vi "DeleteRecord.vi"(0 "reference in":refnum<class "CustomersData.lvclass">, 2 "Customer":string, 5 "error in (no error)":errorcluster) -> (14 "reference out":refnum<class "CustomersData.lvclass">, 19 "error out":errorcluster)   [LabVIEW 2020, in "CustomersData.lvclass"]
uses:
  CustomersData.lvclass
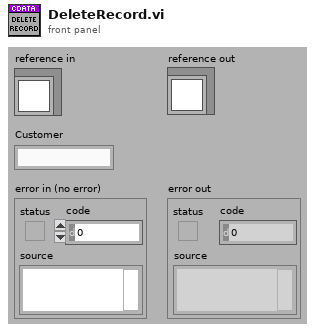
[diagram p1: front panel]
types:
  T1 = typedef "CustomersData.lvclass/ObjectAttributes.ctl" = cluster{"_customers":string[], "_current":i32}
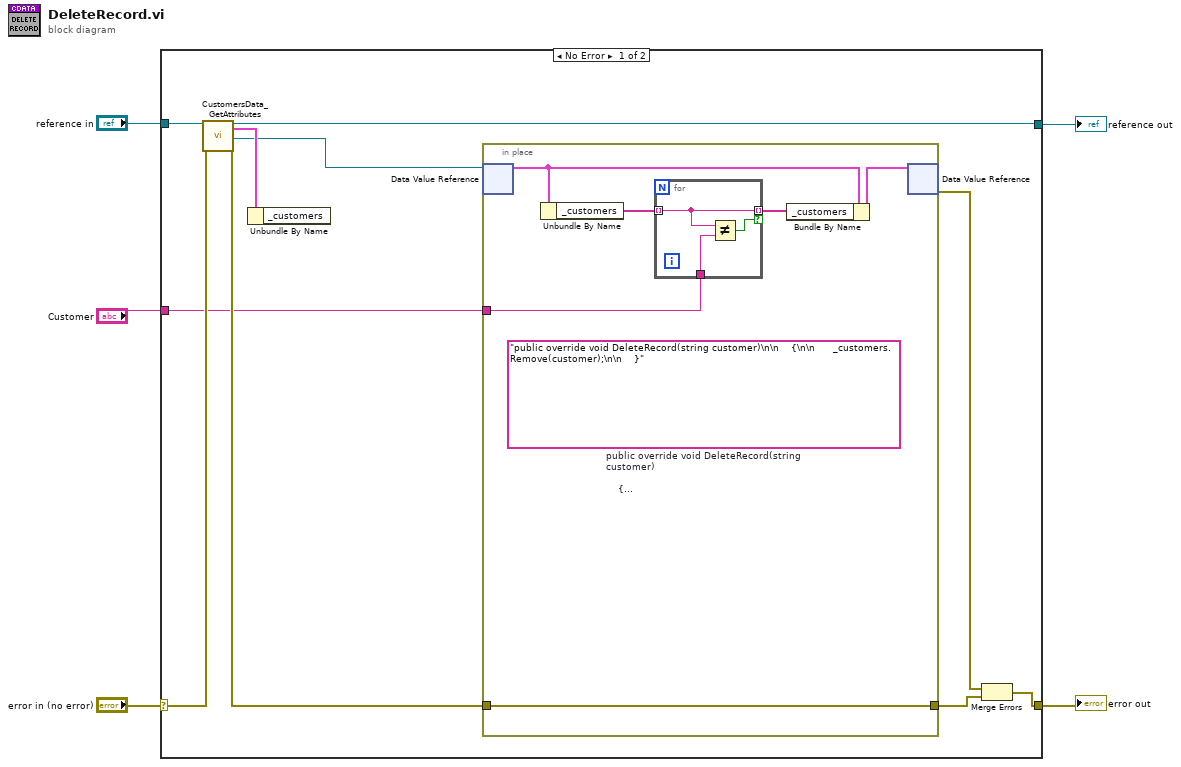
[diagram p0: block diagram]
diagram:
  n1 = case shown="No Error" "error in (no error)" {
    selector: "error in (no error)" -> [w14 w26]
    tunnel: [w11 w26] -> w4
    tunnel: [w10 w25] -> w2
    tunnel: "reference in" -> [w15 w25]
    tunnel: "Customer" -> [w6 _]
    frame No Error {
      n2 = call "CustomersData_GetAttributes.vi"("reference in"=w15, "error in (no error)"=w14) -> ("reference out"=w10:refnum<class "CustomersData.lvclass">, "Data"=w13:T1, "DataRef"=w9:refnum<data-value>, "error out"=w8:errorcluster)  [unwired: 14 in]
      n3 = Unbundle By Name(w13) -> ()  [unwired: 1 out]
      n4 = in-place {
        in-place-border: w8 -> [w20]
        in-place-border: [w20] -> w7
        in-place-border: w6 -> [w17]
        (unwired) "public override void DeleteRecord(string customer)\n\n    {\n\n      _customers.Remove(customer);\n\n    }"  # public override void DeleteRecord(string customer)      {        _customers.Remove(customer);      }
        n5 = in-place-dvr #1(w9) -> (w19:T1)  [unwired: 1 out]
        n6 = Unbundle By Name(w19) -> ("_customers"=w18:string[])
        n7 = for {
          tunnel: w18 -> [w24] mode=indexing
          tunnel: w17 -> [w23]
          tunnel: [w24] -> w16 mode=indexing if=w22
          n8 = Not Equal?(x=w24, y=w23) -> (x != y?=w22:bool)
        }
        n9 = Bundle By Name(cluster=w19, "_customers"=w16) -> (w21:T1)
        n10 = in-place-dvr #1(w21) -> (w12:errorcluster)  [unwired: 1 out]
      }
      n11 = Merge Errors(w12, w7) -> (w11:errorcluster)
    }
    frame Error {
    }
  }
  "error out" <- w4
  "reference out" <- w2
